vi "Restore Input.vi"(0 "VISA resource name":refnum<visa-resource-name>, 1 "Unit Address (1)":i16=1, 5 "Input (1)":i16=1, 11 "error in (no error)":errorcluster {"code" format="%.0x"}) -> (4 "VISA resource name out":refnum<visa-resource-name>, 15 "error out":errorcluster {"code" format="%.0x"})   [LabVIEW 2010]
doc: "This VI restores original factory calibration values."
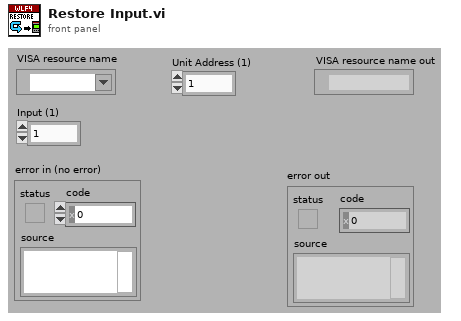
[diagram p1: front panel]
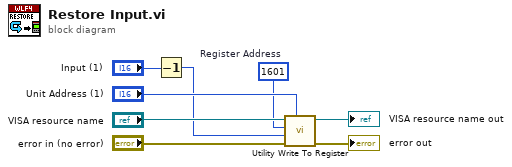
[diagram p0: block diagram]
diagram:
  w3 = u16 1601  # Register Address
  n1 = Decrement(x="Input (1)") -> (x-1=w1:i16)
  n2 = call "Utility Write To Register.vi"("Unit Address (1)"="Unit Address (1)", "error in (no error)"="error in (no error)", "Data (0)"=w1, "Register Address (0)"=w3, "VISA resource name"="VISA resource name") -> ("error out"=→"error out":errorcluster, "VISA resource name out"=→"VISA resource name out":refnum<visa-resource-name>)  [unwired: 5 in]
